vi "theshhold_iter_resetable.vi"(7 "reset":bool, 11 "N":i16) -> (0 "iter":i16, 3 "Boolean":bool)   [LabVIEW 2017, in "libimaging-cs.lvlib"]
doc: "Provides a counter that \nresetts itself ever N iterations.\n\nAt the Nth iteration, the boolean \ntriggers HIGH."
uses:
  libimaging-cs.lvlib
panel:
  # "Provides a counter that \nresetts itself ever N iterations.\n\nAt the Nth iteration, the boolean \ntriggers HIGH."
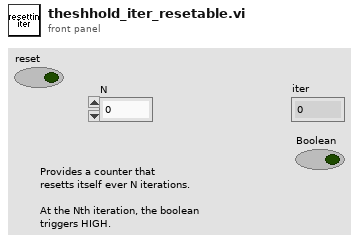
[diagram p1: front panel]
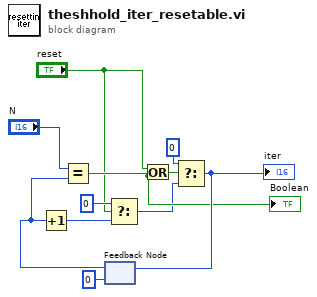
[diagram p0: block diagram]
diagram:
  n1 = feedback #1(i16 0) -> (w10:i16)
  n2 = Increment(x=w10) -> (x+1=w4:i16)
  n3 = Equal?(x="N", y=w10) -> (x = y?=w5:bool)
  "Boolean" <- w5
  n4 = Select(t=i16 0, s="reset", f=w4) -> (s? t:f=w1:i16)
  n5 = Or(x="reset", y=w5) -> (x .or. y?=w6:bool)
  n6 = Select(t=i16 0, s=w6, f=w1) -> (s? t:f=w7:i16)
  "iter" <- w7
  n7 = feedback-in #1(w7) -> ()
